vi "Test Refresh New Active Objects.vi"(8 "error in (no error)":errorcluster) -> (0 "error out":errorcluster)   [LabVIEW 2019]
uses:
  Setting Database/Setting Database.lvclass
  C:/Program Files (x86)/National Instruments/LabVIEW 2019/vi.lib/JKI/JKI SMO/SMO/SMO.lvclass
  <vilib>/addons/_JKI Toolkits/Caraya/classes/Assert/Assert Equal Value_Variant.vi
  <vilib>/addons/_JKI Toolkits/Caraya/classes/Test/Test.lvclass
  <vilib>/addons/_JKI Toolkits/Caraya/classes/Assert/Assert.lvclass
  <vilib>/JKI/JKI SMO/SMO/SMO.lvclass
  <vilib>/LabVIEW Open Source Project/Unicity/RandomStringGenerator/RandomStringGenerator.lvclass
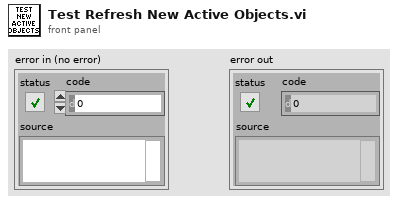
[diagram p1: front panel]
types:
  T1 = typedef "Setting Database.lvclass/PublicEvents--Cluster.ctl" = cluster{"NewActivePath":refnum<user-event>, "PathsUpdated":refnum<user-event>, "RectanglesUpdated":refnum<user-event>, "NewActiveRectangle":refnum<user-event>, "NewActiveFunnel":refnum<user-event>, "FunnelsUpdated":refnum<user-event>, "NewActiveDot":refnum<user-event>, "DotsUpdated":refnum<user-event>}
  T2 = typedef "Setting Database.lvclass/PrivateEvents--Setting Database.Refresh.ctl" = cluster{"Paths":string[], "Rectangles":string[], "Funnels":string[], "Dots":string[]}
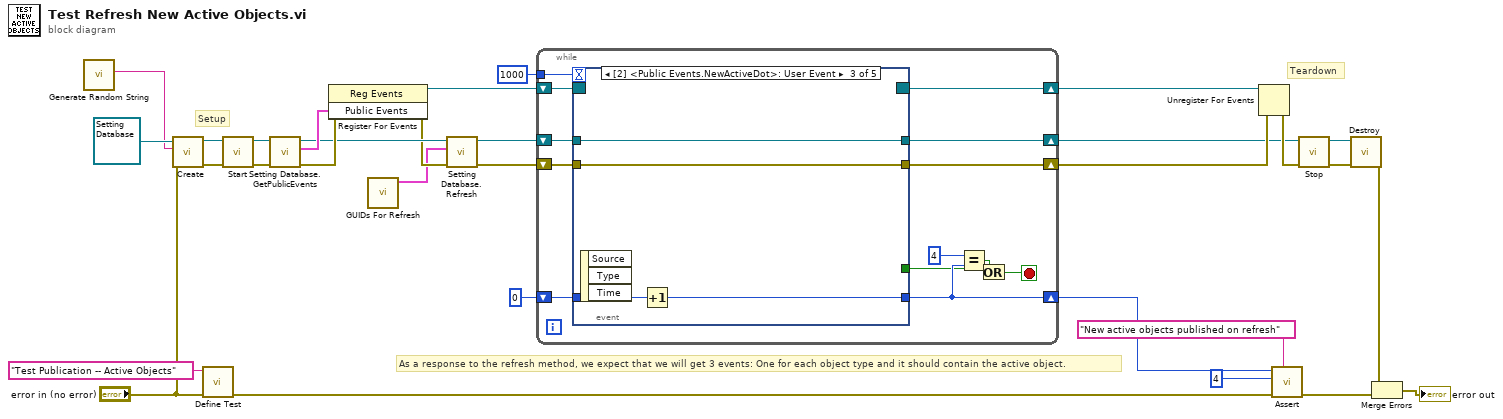
[diagram p0: block diagram]
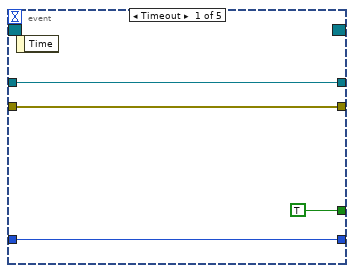
[diagram p2: hidden frame]
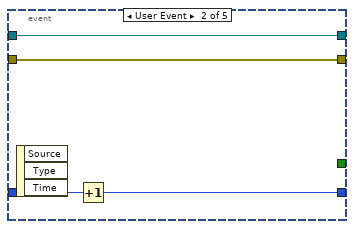
[diagram p3: hidden frame]
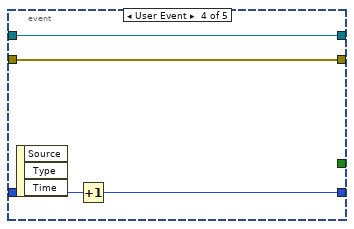
[diagram p4: hidden frame]
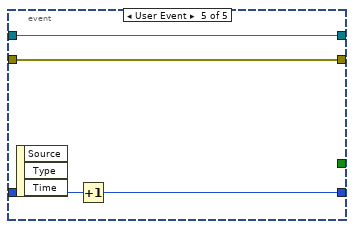
[diagram p5: hidden frame]
diagram:
  # "As a response to the refresh method, we expect that we will get 3 events: One for each object type and it should contain the active object."
  # "Teardown"
  # "Setup"
  n1 = call <vilib>:"Generate Random String.vi"() -> ("Random String"=w1:string)  [unwired: 11 in]
  n2 = call <vilib>:"Create.vi"("error in (no error)"="error in (no error)", "Subsystem Name (optional)"=w1, "SMO"=refnum<class "Setting Database.lvclass"> refnum ("Setting Database.lvclass")) -> ("error out"=w28:errorcluster, "SMO out"=w19:refnum<class "Setting Database.lvclass">)  [unwired: 6 in, 1 out]
  n3 = call <vilib>:"Define Test.vi"("error in (no error)"="error in (no error)", "Label (VI Title)"="Test Publication -- Active Objects") -> ("error out"=w30:errorcluster)  [unwired: 8 in, 1 out]
  n4 = call <vilib>:"Start.vi"("error in (no error)"=w28, "SMO"=w19) -> ("error out"=w27:errorcluster, "SMO out"=w18:refnum<class "Setting Database.lvclass">)  [unwired: 8 in]
  n5 = call "Setting Database.GetPublicEvents.vi"("error in (no error)"=w27, "Setting Database"=w18) -> ("error out"=w24:errorcluster, "Public Events"=w16:T1, "Setting Database out"=w6:refnum<class "Setting Database.lvclass">)  [unwired: 7 in]
  n6 = register-events(error in=w24, w16) -> (reference out=w14:refnum<event-registration>, error out=w4:errorcluster)  [unwired: 1 in]
  n7 = call "GUIDs For Refresh.vi"() -> ("Initialize"=w2:T2)  [unwired: 11 in]
  n8 = call "Setting Database.Refresh.vi"("error in (no error)"=w4, "Initialize"=w2, "Setting Database"=w6) -> ("error out"=w3:errorcluster, "Setting Database out"=w5:refnum<class "Setting Database.lvclass">)  [unwired: 7 in]
  n9 = while {
    shift-right: [w43] -> w11
    shift-left: w14 -> [w42]
    shift-right: [w41] -> w12
    shift-left: w5 -> [w40]
    shift-right: [w44] -> w13
    shift-left: w3 -> [w39]
    shift-right: [w35] -> w8
    shift-left: 0 -> [w38]
    tunnel: 1000 -> [w37]
    stop <- w33 stop-if-true
    n10 = event shown="[2] <Public Events.NewActiveDot>: User Event" {
      selector: w42 -> [_ _ _ _ _]
      dyn-events: [_ _ _ _ _] -> w43
      timeout: w37 -> [_ _ _ _ _]
      tunnel: [w48 w52 w56 w60 w64] -> w44
      tunnel: w39 -> [w48 w52 w56 w60 w64]
      tunnel: w40 -> [w47 w51 w55 w59 w63]
      tunnel: [w47 w51 w55 w59 w63] -> w41
      tunnel: w38 -> [w46 w50 w54 w58 w62]
      tunnel: [w46 w49 w53 w57 w61] -> w35
      tunnel: [TRUE _ _ _ _] -> w32
      event Timeout {
        n11 = event-data() -> ()  [unwired: 1 in, 1 out]
      }
      event User Event {
        n12 = event-data() -> ()  [unwired: 1 in, 3 out]
        n13 = Increment(x=w50) -> (x+1=w49:i32)
      }
      event User Event {
        n14 = event-data() -> ()  [unwired: 1 in, 3 out]
        n15 = Increment(x=w54) -> (x+1=w53:i32)
      }
      event User Event {
        n16 = event-data() -> ()  [unwired: 1 in, 3 out]
        n17 = Increment(x=w58) -> (x+1=w57:i32)
      }
      event User Event {
        n18 = event-data() -> ()  [unwired: 1 in, 3 out]
        n19 = Increment(x=w62) -> (x+1=w61:i32)
      }
    }
    n20 = Equal?(x=4, y=w35) -> (x = y?=w34:bool)
    n21 = Or(x=w32, y=w34) -> (x .or. y?=w33:bool)
  }
  n22 = Unregister For Events(event registration refnum=w11, error in=w13) -> (error out=w25:errorcluster)
  n23 = call-poly <vilib>:"Assert.vi"("Label"="New active objects published on refresh" ("Label (VI Title)"), "error in (no error)"=w30, "Actual"=4, "Expected"=w8) -> ("error out"=w31:errorcluster)  [unwired: 6 in, 1 out]
  n24 = call <vilib>:"Stop.vi"("error in (no error)"=w25, "SMO"=w12) -> ("error out"=w26:errorcluster, "SMO out"=w17:refnum<class "Setting Database.lvclass">)  [unwired: 8 in]
  n25 = call <vilib>:"Destroy.vi"("error in (no error)"=w26, "SMO"=w17) -> ("error out"=w23:errorcluster)  [unwired: 9 in]
  n26 = Merge Errors(w23, w31) -> (→"error out":errorcluster)
